vi "Configure Sensitivity and Reserve.vi"(8 "error in (no error)":errorcluster, 9 "Sensitivity (-1: Auto gain)":i16(ring)=-1 items=["Auto Gain"=-1, "2 nV/fA"=0, "5 nV/fA"=1, "10 nV/fA"=2, "20 nV/fA"=3, "50 nV/fA"=4, "100 nV/fA"=5, "200 nV/fA"=6, "500 nV/fA"=7, "1 uV/pA"=8, "2 uV/pA"=9, "5 uV/pA"=10, "10 uV/pA"=11, "20 uV/pA"=12, "50 uV/pA"=13, "100 uV/pA"=14, "200 uV/pA"=15, "500 uV/pA"=16, "1 mV/nA"=17, "2 mV/nA"=18, "5 mV/nA"=19, "10 mV/nA"=20, "20 mV/nA"=21, "50 mV/nA"=22, "100 mV/nA"=23, "200 mV/nA"=24, "500 mV/mA"=25, "1 V/uA"=26], 10 "Dynamic Reserve (-1: Auto Reserve)":i16(ring)=-1 items=["Auto Reserve"=-1, "High Reserve"=0, "Normal"=1, "Low Noise"=2], 11 "VISA resource name":refnum<visa-resource-name>) -> (0 "error out":errorcluster, 3 "VISA resource name out":refnum<visa-resource-name>)   [LabVIEW 2012, in "Stanford Research 830.lvlib"]
doc: "Configures the instrument's dynamic reserve and sensitivity."
uses:
  Stanford Research 830.lvlib
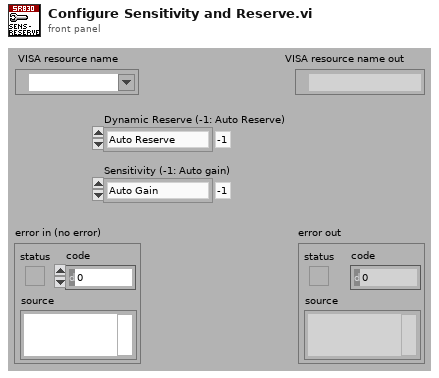
[diagram p1: front panel]
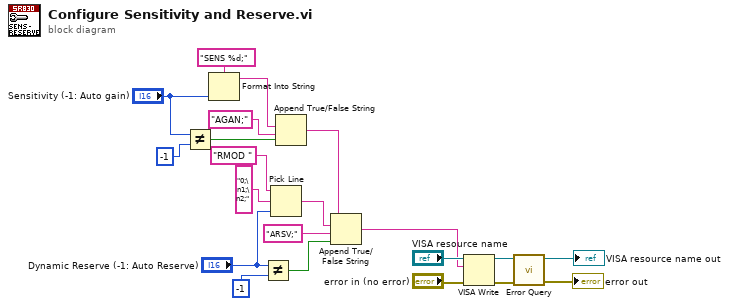
[diagram p0: block diagram]
diagram:
  n1 = Not Equal?(x="Sensitivity (-1: Auto gain)", y=i16 -1) -> (x != y?=w9:bool)
  n2 = Format Into String(format string="SENS %d;", "Sensitivity (-1: Auto gain)") -> (resulting string=w8:string)  [unwired: 2 in, 1 out]
  n3 = Not Equal?(x="Dynamic Reserve (-1: Auto Reserve)", y=i16 -1) -> (x != y?=w19:bool)
  n4 = Pick Line(string ("")="RMOD ", multi-line string="0;\n1;\n2;", line index="Dynamic Reserve (-1: Auto Reserve)") -> (output string=w14:string)
  n5 = Append True/False String(1:w9, 2:"AGAN;" ("false string"), 3:w8) -> (0:w6:string)  [unwired: 1 in]
  n6 = Append True/False String(1:w19, 2:"ARSV;" ("false string"), 3:w14, 4:w6) -> (0:w5:string)
  n7 = VISA Write(VISA resource name="VISA resource name", write buffer=w5, error in (no error)="error in (no error)") -> (VISA resource name out=w4:refnum<visa-resource-name>, error out=w1:errorcluster)  [unwired: 1 out]
  n8 = call "Error Query.vi"("error in (no error)"=w1, "VISA resource name"=w4) -> ("error out"=→"error out":errorcluster, "VISA resource name out"=→"VISA resource name out":refnum<visa-resource-name>)  [unwired: 7 in, 1 out]
